vi "Read Input Module.vi"(4 "IOV ref":refnum<k21>, 5 "Channel Type":T6, 6 "Model":T1, 7 "R/W Case":T2, 8 "error in (no error)":errorcluster, 9 "Output FIFO buffer in":dbl[](array[numeric]), 10 "Output Data in":T3 {"BD Refs"."Data Reference" format="%.0x"}, 11 "IOV ref in":T7) -> (0 "error out":errorcluster, 1 "Output FIFO buffer out":dbl[](array[numeric]), 2 "Output Data out":T3 {"BD Refs"."Data Reference" format="%.0x"}, 3 "IOV ref out":T7)   [LabVIEW 2016, in "Scan Engine Custom Device.lvlib"]
uses:
  Scan Engine Custom Device.lvlib
  <vilib>/NI Veristand/Custom Device API/Custom Device API.lvlib
  <vilib>/NI Veristand/Custom Device API/Data Reference.ctl
  <vilib>/NI Veristand/Custom Device API/Block Data Reference.ctl
  Type Defs/Output Data.ctl
  Modules.lvlibp/RSI Module/Channel Type.ctl
  Type Defs/RW Case.ctl
  Type Defs/Open Module IOVs.ctl
  Modules.lvlibp/RSI Module/Module Models.ctl
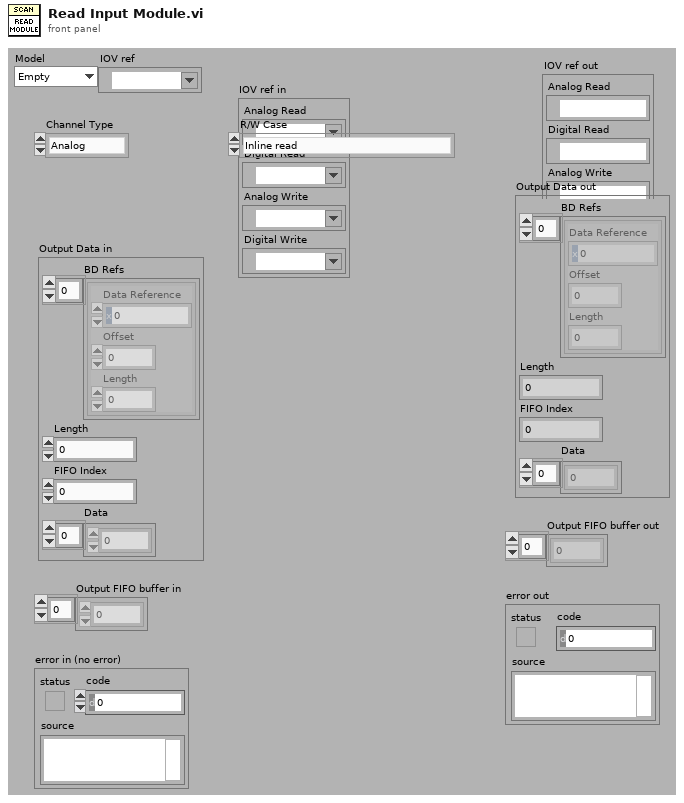
[diagram p1: front panel]
types:
  T1 = typedef "Modules.lvlibp/RSI Module.lvclass/Module Models.ctl" = enum16{"Empty", "NI 9201", "NI 9203", "NI 9205", "NI 9206", "NI 9207", "NI 9208", "NI 9211", "NI 9213", "NI 9214", "NI 9215", "NI 9217", "NI 9219", "NI 9221", "NI 9225", "NI 9227", "NI 9229", "NI 9233", "NI 9234", "NI 9235", "NI 9236", "NI 9237", "NI 9239", "NI 9263", "NI 9264", "NI 9265", "NI 9269", "NI 9375", "NI 9401", "NI 9402", "NI 9403", "NI 9411", "NI 9421", "NI 9422", "NI 9423", "NI 9425", "NI 9426", "NI 9435", "NI 9472", "NI 9474", "NI 9475", "NI 9476", "NI 9477", "NI 9478", "NI 9481", "NI 9482", "NI 9485"}
  T2 = typedef "Scan Engine Custom Device.lvlib/RW Case.ctl" = enum16{"Inline read", "Inline write", "Async - Inline loop read", "Async - Inline loop write", "Async loop (read/write)"}
  T3 = typedef "Scan Engine Custom Device.lvlib/Output Data.ctl" = cluster{"BD Refs":T4[], "Length":i32, "FIFO Index":i32, "Data":dbl[]}
  T4 = typedef "Custom Device API.lvlib/Block Data Reference.ctl" = cluster{"Data Reference":T5, "Offset":u64, "Length":u64}
  T5 = typedef "Custom Device API.lvlib/Data Reference.ctl" = i32
  T6 = typedef "Modules.lvlibp/RSI Module.lvclass/Channel Type.ctl" = enum16{"Analog", "Digital"}
  T7 = typedef "Scan Engine Custom Device.lvlib/Open Module IOVs.ctl" = cluster{"Analog Read":refnum<k21>, "Digital Read":refnum<k21>, "Analog Write":refnum<k21>, "Digital Write":refnum<k21>}
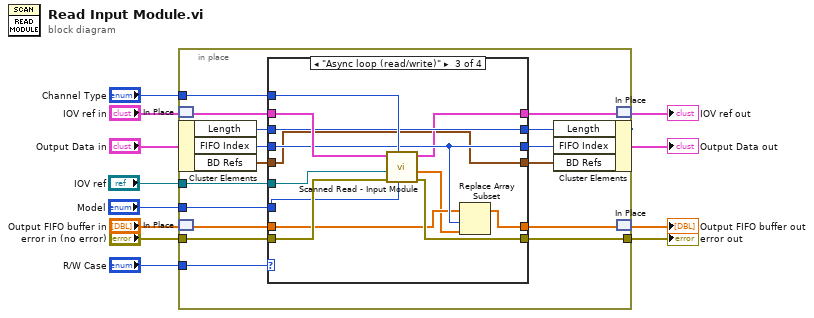
[diagram p0: block diagram]
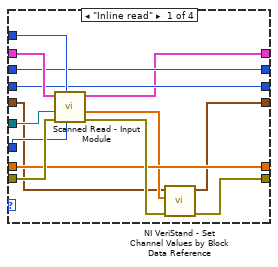
[diagram p2: hidden frame]
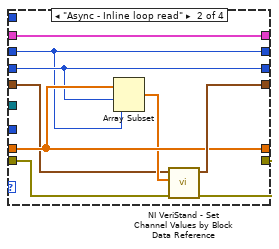
[diagram p3: hidden frame]
diagram:
  n1 = in-place {
    in-place-border: "R/W Case" -> [w28]
    in-place-border: "Channel Type" -> [w27]
    in-place-border: "error in (no error)" -> [w26]
    in-place-border: [w24] -> w6
    in-place-border: "Model" -> [w14]
    in-place-border: "IOV ref" -> [w13]
    n2 = in-place-match #1("IOV ref in") -> (w16:T7)
    n3 = in-place-cluster #2("Output Data in") -> ("Length"=w19:i32, "FIFO Index"=w22:i32, "BD Refs"=w25:T4[])
    n4 = in-place-match #3("Output FIFO buffer in") -> (w18:dbl[])
    n5 = case shown="\"Async loop (read/write)\"" w28 {
      tunnel: w27 -> [w42 _ w64 _]
      tunnel: w16 -> [w41 w45 w63 w70]
      tunnel: w26 -> [w40 w51 w62 w65]
      tunnel: w18 -> [w34 w48 w57 w66]
      tunnel: w25 -> [w29 w43 w56 w67]
      tunnel: [w35 w50 w58 w65] -> w24
      tunnel: [w33 w49 w56 w67] -> w23
      tunnel: [w34 w48 w55 w66] -> w17
      tunnel: w22 -> [w39 w47 w61 w68]
      tunnel: [w39 w47 w61 w68] -> w21
      tunnel: [w38 w46 w60 w69] -> w20
      tunnel: [w37 w45 w59 w70] -> w15
      tunnel: w19 -> [w38 w46 w60 w69]
      tunnel: w14 -> [w32 _ w53 _]
      tunnel: w13 -> [w31 _ w52 _]
      frame "Inline read" {
        n6 = call "Scanned Read - Input Module.vi"("Model"=w32, "Channel Type"=w42, "error in (no error)"=w40, "IOV ref"=w31, "IOV ref in"=w41) -> ("error out"=w36:errorcluster, "channel data"=w30:dbl[], "IOV ref out"=w37:T7)  [unwired: 4 in]
        n7 = call <vilib>:"NI VeriStand - Set Channel Values by Block Data Reference.vi"("error in (no error)"=w36, "Values Array in"=w30, "Block Data Ref"=w29) -> ("error out"=w35:errorcluster, "Block Data Ref dup"=w33:T4[])  [unwired: 6 in, 1 out]
      }
      frame "Async - Inline loop read" {
        n8 = Array Subset(array=w48, index=w47, length=w46) -> (w44:dbl[])
        n9 = call <vilib>:"NI VeriStand - Set Channel Values by Block Data Reference.vi"("error in (no error)"=w51, "Values Array in"=w44, "Block Data Ref"=w43) -> ("error out"=w50:errorcluster, "Block Data Ref dup"=w49:T4[])  [unwired: 6 in, 1 out]
      }
      frame "Async loop (read/write)" {
        n10 = call "Scanned Read - Input Module.vi"("Model"=w53, "Channel Type"=w64, "error in (no error)"=w62, "IOV ref"=w52, "IOV ref in"=w63) -> ("error out"=w58:errorcluster, "channel data"=w54:dbl[], "IOV ref out"=w59:T7)  [unwired: 4 in]
        n11 = Replace Array Subset(array=w57, new element=w54, index=w61) -> (w55:dbl[])
      }
      frame Default {
      }
    }
    n12 = in-place-cluster #2("Length"=w20, "FIFO Index"=w21, "BD Refs"=w23) -> (→"Output Data out":T3)
    n13 = in-place-match #1(w15) -> (→"IOV ref out":T7)
    n14 = in-place-match #3(w17) -> (→"Output FIFO buffer out":dbl[])
  }
  "error out" <- w6
